vi "Set Help Document Display.vi"(8 "error in (no error)":errorcluster, 9 "HTML File to Load":string, 11 "SHDocVw.IWebBrowser2":refnum<k7>(container)) -> (0 "error out":errorcluster)   [LabVIEW 2020, in "SLSC-12201 DIO System Explorer.lvlib"]
uses:
  SLSC-12201 DIO System Explorer.lvlib
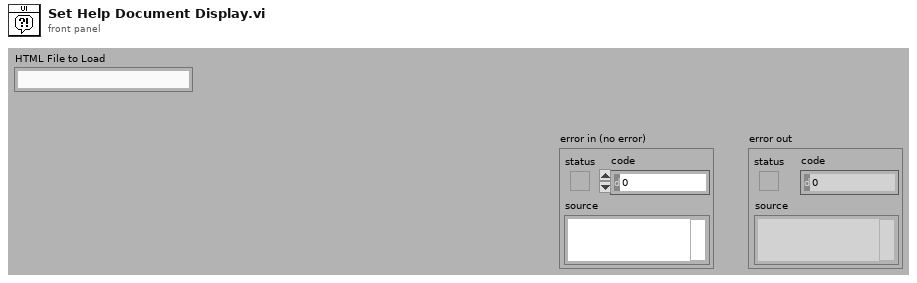
[diagram p1: front panel]
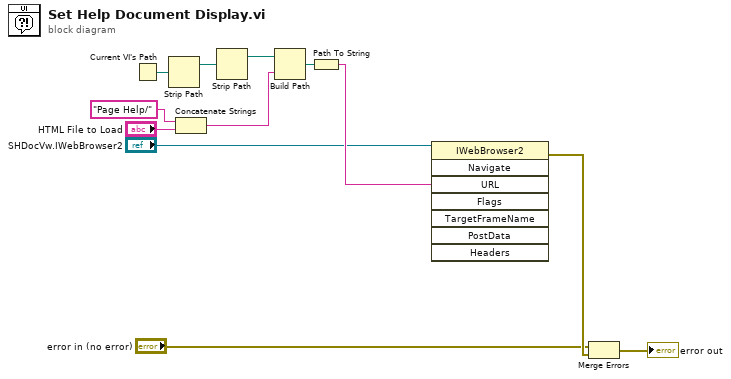
[diagram p0: block diagram]
diagram:
  n1 = Current VI's Path() -> (path=w12:path)
  n2 = Strip Path(path=w12) -> (stripped path=w11:path)  [unwired: 1 out]
  n3 = Concatenate Strings("Page Help/" ("string"), "HTML File to Load") -> (w2:string)
  n4 = Strip Path(path=w11) -> (stripped path=w7:path)  [unwired: 1 out]
  n5 = Build Path(base path=w7, name or relative path=w2) -> (appended path=w9:path)
  n6 = Path To String(path=w9) -> (string=w10:string)
  n7 = invoke class="IWebBrowser2" method="Navigate"(reference="SHDocVw.IWebBrowser2", "URL"=w10) -> (error out=w5:errorcluster)  [unwired: 6 in, 7 out]
  n8 = Merge Errors("error in (no error)", w5) -> (→"error out":errorcluster)
